vi "Run.vi"(8 "error in (no error)":errorcluster, 11 "SecMirror in":refnum<class "SecMirror.lvclass">) -> (0 "error out":errorcluster, 3 "SecMirror out":refnum<class "SecMirror.lvclass">)   [LabVIEW 2018, in "SecMirror.lvclass"]
uses:
  SecMirror.lvclass
  SecMirror.lvclass/SecMirror.ctl
  Device/Device.lvclass
  StateMachine/State Machine.lvclass
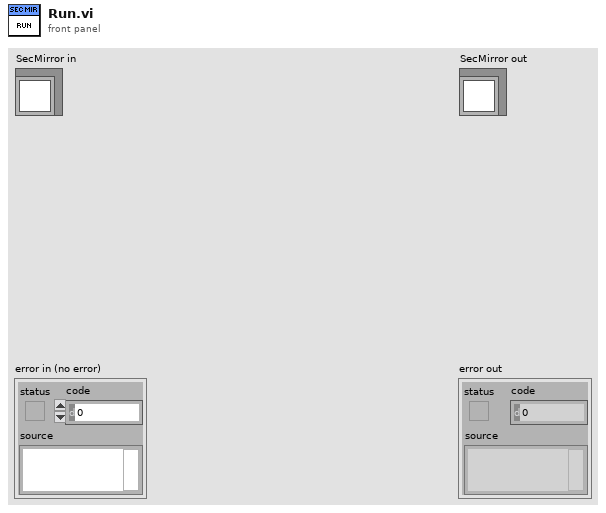
[diagram p1: front panel]
types:
  T1 = cluster{"clientId":string, "clientTransactionId":string, "clientName":string, "action":string}
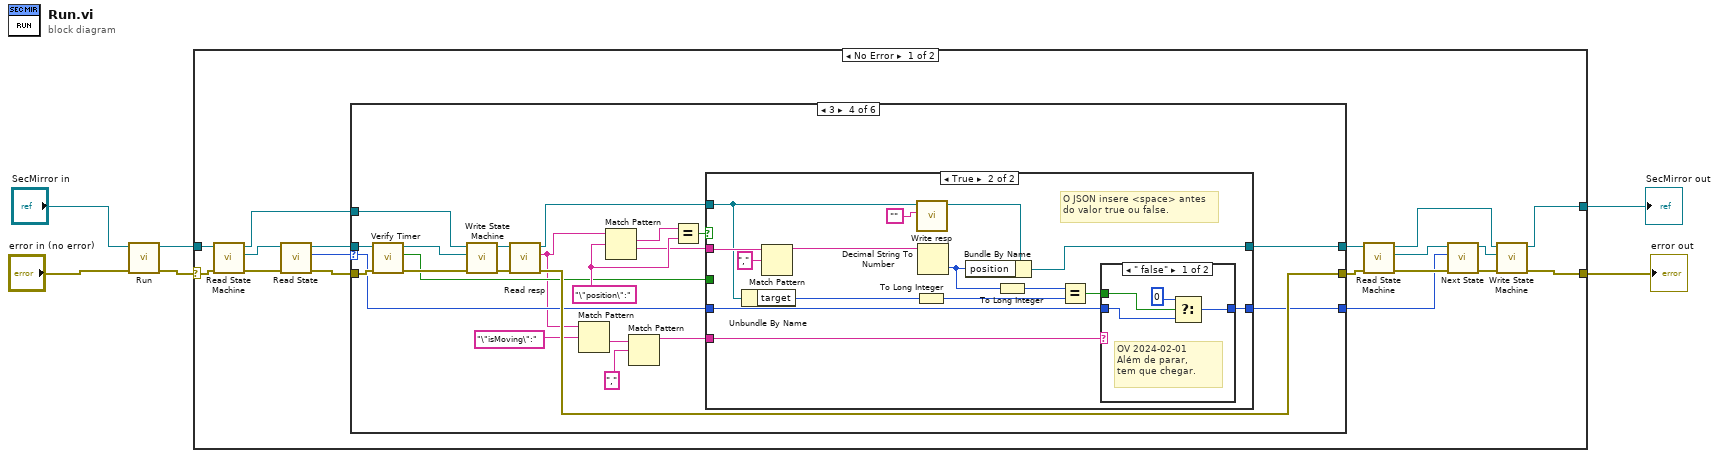
[diagram p0: block diagram]
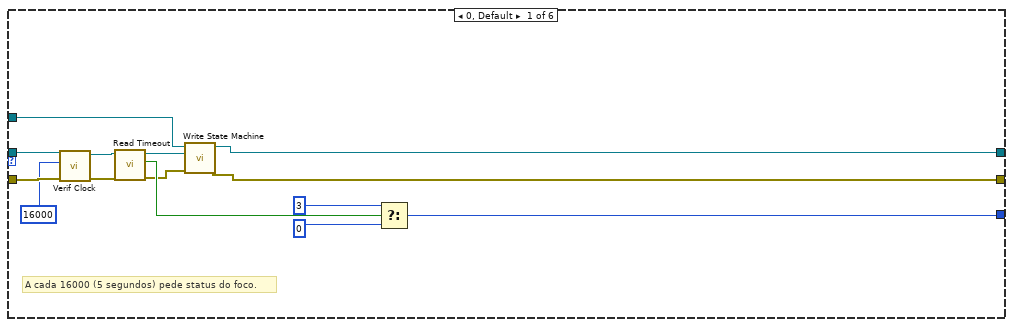
[diagram p2: hidden frame]
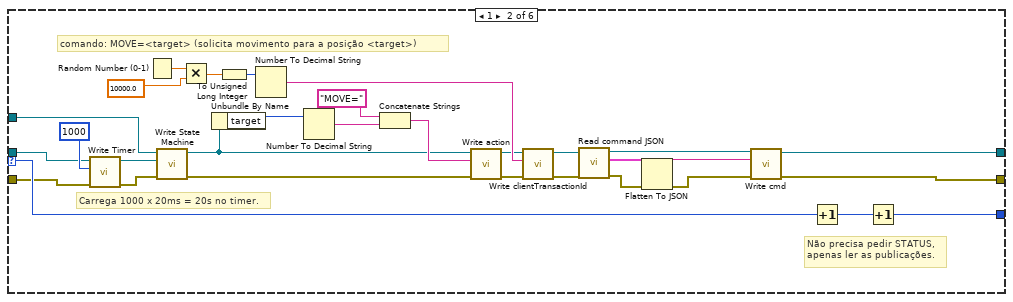
[diagram p3: hidden frame]
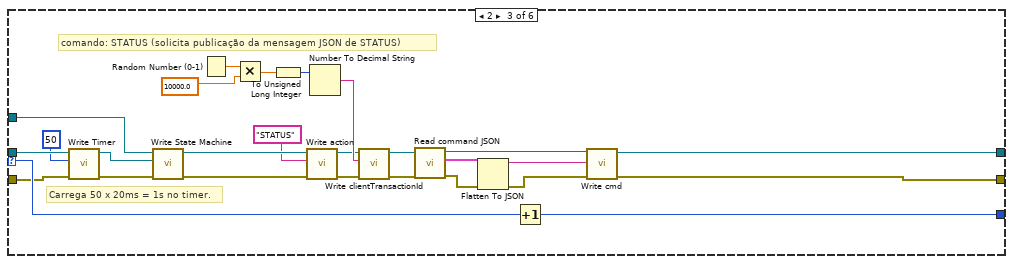
[diagram p4: hidden frame]
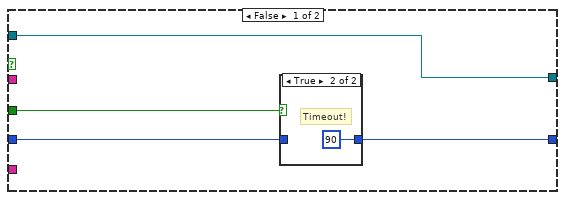
[diagram p5: hidden frame]
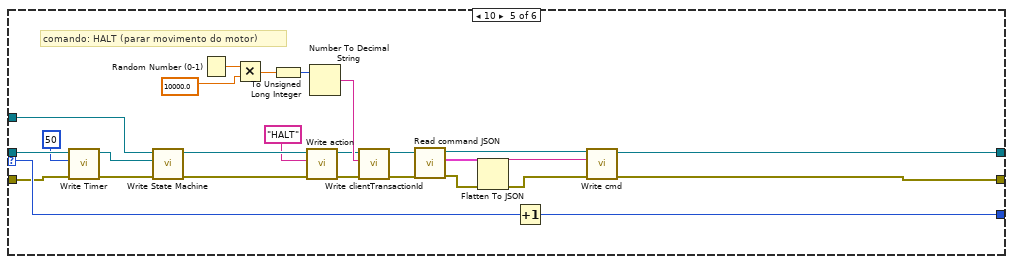
[diagram p8: hidden frame]
diagram:
  n1 = call-parent "Run.vi"("error in (no error)"="error in (no error)", "Device in"="SecMirror in") -> ("error out"=w3:errorcluster, "Device out"=w4:refnum<class "SecMirror.lvclass">)  [unwired: 8 in]
  n2 = case shown="No Error" w3 {
    selector: w3 -> [w23 w176]
    tunnel: [w15 w176] -> w1
    tunnel: w4 -> [w24 w175]
    tunnel: [w14 w175] -> w2
    frame No Error {
      n3 = call-dynamic "Read State Machine.vi"("error in (no error)"=w23, "Device in"=w24) -> ("error out"=w21:errorcluster, "State Machine.lvclass"=w22:refnum<class "State Machine.lvclass">, "Device out"=w12:refnum<class "SecMirror.lvclass">)  [unwired: 7 in]
      n4 = call-dynamic "Read State.vi"("error in (no error)"=w21, "State Machine in"=w22) -> ("error out"=w11:errorcluster, "State"=w13:i32, "State Machine out"=w7:refnum<class "State Machine.lvclass">)  [unwired: 7 in]
      n5 = case shown="3" w13 {
        selector: w13 -> [_ w69 w96 w107 w171 w172]
        tunnel: w12 -> [w30 w46 w92 w112 w167 w174]
        tunnel: w11 -> [w33 w44 w91 w110 w166 w173]
        tunnel: [w26 w39 w70 w116 w145 w173] -> w10
        tunnel: [w27 w40 w71 w117 w146 w174] -> w9
        tunnel: [w38 w49 w95 w115 w170 w172] -> w8
        tunnel: w7 -> [w32 w47 w94 w114 w169 _]
        frame 0, Default {
          # "A cada 16000 (5 segundos) pede status do foco."
          n6 = call-dynamic "Verif Clock.vi"("error in (no error)"=w33, "period (ms)"=u32 16000 ("period"), "State Machine in"=w32) -> ("error out"=w34:errorcluster, "State Machine out"=w31:refnum<class "State Machine.lvclass">)  [unwired: 6 in, 1 out]
          n7 = call-dynamic "Read Timeout.vi"("error in (no error)"=w34, "State Machine in"=w31) -> ("error out"=w28:errorcluster, "Timeout"=w35:bool, "State Machine out"=w29:refnum<class "State Machine.lvclass">)  [unwired: 7 in]
          n8 = call-dynamic "Write State Machine.vi"("error in (no error)"=w28, "State Machine.lvclass"=w29, "Device in"=w30) -> ("error out"=w26:errorcluster, "Device out"=w27:refnum<class "SecMirror.lvclass">)  [unwired: 7 in]
          n9 = Select(t=3 ("State"), s=w35, f=0 ("State")) -> (s? t:f=w38:i32)
        }
        frame 1 {
          # "Carrega 1000 x 20ms = 20s no timer."
          # "Não precisa pedir STATUS,\napenas ler as publicações."
          # "comando: MOVE=<target> (solicita movimento para a posição <target>)"
          n10 = call-dynamic "Write Timer.vi"("error in (no error)"=w44, "Timer"=u32 1000, "State Machine in"=w47) -> ("error out"=w43:errorcluster, "State Machine out"=w42:refnum<class "State Machine.lvclass">)  [unwired: 7 in]
          n11 = Random Number (0-1)() -> (number: 0 to 1=w64:dbl)
          n12 = call-dynamic "Write State Machine.vi"("error in (no error)"=w43, "State Machine.lvclass"=w42, "Device in"=w46) -> ("error out"=w41:errorcluster, "Device out"=w45:refnum<class "SecMirror.lvclass">)  [unwired: 7 in]
          n13 = Multiply(x=w64, y=10000.0) -> (x*y=w61:dbl)
          n14 = Unbundle By Name(w45) -> ("target"=w66:i32)
          n15 = To Unsigned Long Integer(number=w61) -> (unsigned 32bit integer=w60:u32)
          n16 = Number To Decimal String(number=w60) -> (decimal integer string=w59:string)  [unwired: 1 in]
          n17 = Number To Decimal String(number=w66) -> (decimal integer string=w65:string)  [unwired: 1 in]
          n18 = Concatenate Strings("MOVE=" ("cmd"), w65) -> (w63:string)
          n19 = call-dynamic "Write action.vi"("error in (no error)"=w41, "action"=w63, "Device in"=w45) -> ("error out"=w57:errorcluster, "Device out"=w58:refnum<class "SecMirror.lvclass">)  [unwired: 7 in]
          n20 = call-dynamic "Write clientTransactionId.vi"("error in (no error)"=w57, "clientTransactionId"=w59, "Device in"=w58) -> ("error out"=w55:errorcluster, "Device out"=w56:refnum<class "SecMirror.lvclass">)  [unwired: 7 in]
          n21 = call-dynamic "Read command JSON.vi"("error in (no error)"=w55, "Device in"=w56) -> ("error out"=w53:errorcluster, "command JSON"=w54:T1, "Device out"=w52:refnum<class "SecMirror.lvclass">)  [unwired: 7 in]
          n22 = Flatten To JSON(anything=w54, error in (no error)=w53) -> (JSON string=w50:string, 11:w51:errorcluster)  [unwired: 1 in]
          n23 = call-dynamic "Write cmd.vi"("error in (no error)"=w51, "cmd"=w50, "Device in"=w52) -> ("error out"=w39:errorcluster, "Device out"=w40:refnum<class "SecMirror.lvclass">)  [unwired: 7 in]
          n24 = Increment(x=w69) -> (x+1=w68:i32)
          n25 = Increment(x=w68) -> (x+1=w49:i32)
        }
        frame 2 {
          # "Carrega 50 x 20ms = 1s no timer."
          # "comando: STATUS (solicita publicação da mensagem JSON de STATUS)"
          n26 = call-dynamic "Write Timer.vi"("error in (no error)"=w91, "Timer"=u32 50, "State Machine in"=w94) -> ("error out"=w90:errorcluster, "State Machine out"=w89:refnum<class "State Machine.lvclass">)  [unwired: 7 in]
          n27 = call-dynamic "Write State Machine.vi"("error in (no error)"=w90, "State Machine.lvclass"=w89, "Device in"=w92) -> ("error out"=w74:errorcluster, "Device out"=w73:refnum<class "SecMirror.lvclass">)  [unwired: 7 in]
          n28 = Random Number (0-1)() -> (number: 0 to 1=w88:dbl)
          n29 = Multiply(x=w88, y=10000.0) -> (x*y=w86:dbl)
          n30 = To Unsigned Long Integer(number=w86) -> (unsigned 32bit integer=w85:u32)
          n31 = call-dynamic "Write action.vi"("error in (no error)"=w74, "action"="STATUS" ("cmd"), "Device in"=w73) -> ("error out"=w82:errorcluster, "Device out"=w83:refnum<class "SecMirror.lvclass">)  [unwired: 7 in]
          n32 = Number To Decimal String(number=w85) -> (decimal integer string=w84:string)  [unwired: 1 in]
          n33 = call-dynamic "Write clientTransactionId.vi"("error in (no error)"=w82, "clientTransactionId"=w84, "Device in"=w83) -> ("error out"=w80:errorcluster, "Device out"=w81:refnum<class "SecMirror.lvclass">)  [unwired: 7 in]
          n34 = call-dynamic "Read command JSON.vi"("error in (no error)"=w80, "Device in"=w81) -> ("error out"=w78:errorcluster, "command JSON"=w79:T1, "Device out"=w77:refnum<class "SecMirror.lvclass">)  [unwired: 7 in]
          n35 = Flatten To JSON(anything=w79, error in (no error)=w78) -> (JSON string=w75:string, 11:w76:errorcluster)  [unwired: 1 in]
          n36 = Increment(x=w96) -> (x+1=w95:i32)
          n37 = call-dynamic "Write cmd.vi"("error in (no error)"=w76, "cmd"=w75, "Device in"=w77) -> ("error out"=w70:errorcluster, "Device out"=w71:refnum<class "SecMirror.lvclass">)  [unwired: 7 in]
        }
        frame 3 {
          w104 = "\"position\":" ("regular expression")
          n38 = call "Verify Timer.vi"("error in (no error)"=w110, "State Machine in"=w114) -> ("error out"=w111:errorcluster, "timeout"=w103:bool, "State Machine out"=w113:refnum<class "State Machine.lvclass">)  [unwired: 7 in]
          n39 = call-dynamic "Write State Machine.vi"("error in (no error)"=w111, "State Machine.lvclass"=w113, "Device in"=w112) -> ("error out"=w108:errorcluster, "Device out"=w109:refnum<class "SecMirror.lvclass">)  [unwired: 7 in]
          n40 = call-dynamic "Read resp.vi"("error in (no error)"=w108, "Device in"=w109) -> ("error out"=w116:errorcluster, "resp"=w101:string, "Device out"=w118:refnum<class "SecMirror.lvclass">)  [unwired: 7 in]
          n41 = Match Pattern(string=w101, regular expression="\"isMoving\":") -> (after substring=w98:string)  [unwired: 1 in, 3 out]
          n42 = Match Pattern(string=w101, regular expression=w104) -> (match substring=w105:string, after substring=w102:string)  [unwired: 1 in, 2 out]
          n43 = Match Pattern(string=w98, regular expression=",") -> (before substring=w97:string)  [unwired: 1 in, 3 out]
          n44 = Equal?(x=w105, y=w104) -> (x = y?=w106:bool)
          n45 = case shown="True" w106 {
            tunnel: w118 -> [w122 w130]
            tunnel: [w122 w138] -> w117
            tunnel: [w120 w139] -> w115
            tunnel: w107 -> [w121 w131]
            tunnel: w103 -> [w119 _]
            tunnel: w102 -> [_ w134]
            tunnel: w97 -> [_ w132]
            frame False {
              n46 = case shown="True" w119 {
                tunnel: w121 -> [w123 _]
                tunnel: [w123 90 ("State")] -> w120
                frame False {
                }
                frame True {
                  # "Timeout!"
                }
              }
            }
            frame True {
              # "O JSON insere <space> antes\ndo valor true ou false."
              n47 = Unbundle By Name(w130) -> ("target"=w128:i32)
              n48 = Match Pattern(string=w134, regular expression=",") -> (before substring=w133:string)  [unwired: 1 in, 3 out]
              n49 = To Long Integer(number=w128) -> (32bit integer=w125:i32)
              n50 = call-dynamic "Write resp.vi"("resp"="", "Device in"=w130) -> ("Device out"=w137:refnum<class "SecMirror.lvclass">)  [unwired: 8 in, 1 out]
              n51 = Decimal String To Number(string=w133) -> (number=w129:i32)  [unwired: 2 in, 1 out]
              n52 = Bundle By Name(cluster=w137, "position"=w129) -> (w138:refnum<class "SecMirror.lvclass">)
              n53 = To Long Integer(number=w129) -> (32bit integer=w126:i32)
              n54 = Equal?(x=w126, y=w125) -> (x = y?=w127:bool)
              n55 = case shown="\" false\"" w132 {
                tunnel: [w140 w144] -> w139
                tunnel: w131 -> [w141 w144]
                tunnel: w127 -> [w142 _]
                frame " false" {
                  # "OV 2024-02-01\nAlém de parar,\ntem que chegar."
                  n56 = Select(t=0, s=w142, f=w141) -> (s? t:f=w140:i32)
                }
                frame " true", Default {
                }
              }
            }
          }
        }
        frame 10 {
          # "comando: HALT (parar movimento do motor)"
          n57 = call-dynamic "Write Timer.vi"("error in (no error)"=w166, "Timer"=u32 50, "State Machine in"=w169) -> ("error out"=w165:errorcluster, "State Machine out"=w164:refnum<class "State Machine.lvclass">)  [unwired: 7 in]
          n58 = call-dynamic "Write State Machine.vi"("error in (no error)"=w165, "State Machine.lvclass"=w164, "Device in"=w167) -> ("error out"=w149:errorcluster, "Device out"=w148:refnum<class "SecMirror.lvclass">)  [unwired: 7 in]
          n59 = Random Number (0-1)() -> (number: 0 to 1=w163:dbl)
          n60 = Multiply(x=w163, y=10000.0) -> (x*y=w161:dbl)
          n61 = To Unsigned Long Integer(number=w161) -> (unsigned 32bit integer=w160:u32)
          n62 = call-dynamic "Write action.vi"("error in (no error)"=w149, "action"="HALT" ("cmd"), "Device in"=w148) -> ("error out"=w157:errorcluster, "Device out"=w158:refnum<class "SecMirror.lvclass">)  [unwired: 7 in]
          n63 = Number To Decimal String(number=w160) -> (decimal integer string=w159:string)  [unwired: 1 in]
          n64 = call-dynamic "Write clientTransactionId.vi"("error in (no error)"=w157, "clientTransactionId"=w159, "Device in"=w158) -> ("error out"=w155:errorcluster, "Device out"=w156:refnum<class "SecMirror.lvclass">)  [unwired: 7 in]
          n65 = call-dynamic "Read command JSON.vi"("error in (no error)"=w155, "Device in"=w156) -> ("error out"=w153:errorcluster, "command JSON"=w154:T1, "Device out"=w152:refnum<class "SecMirror.lvclass">)  [unwired: 7 in]
          n66 = Flatten To JSON(anything=w154, error in (no error)=w153) -> (JSON string=w150:string, 11:w151:errorcluster)  [unwired: 1 in]
          n67 = Increment(x=w171) -> (x+1=w170:i32)
          n68 = call-dynamic "Write cmd.vi"("error in (no error)"=w151, "cmd"=w150, "Device in"=w152) -> ("error out"=w145:errorcluster, "Device out"=w146:refnum<class "SecMirror.lvclass">)  [unwired: 7 in]
        }
        frame 90 {
          # "Situacao de erro: O focalizador do 1.60 nao publicou o STATUS por 100 x 20m = 2s (estado 1)"
        }
      }
      n69 = call-dynamic "Read State Machine.vi"("error in (no error)"=w10, "Device in"=w9) -> ("error out"=w17:errorcluster, "State Machine.lvclass"=w19:refnum<class "State Machine.lvclass">, "Device out"=w18:refnum<class "SecMirror.lvclass">)  [unwired: 7 in]
      n70 = call "Next State.vi"("error in (no error)"=w17, "New_State"=w8, "State Machine in"=w19) -> ("error out"=w16:errorcluster, "State Machine out"=w20:refnum<class "State Machine.lvclass">)  [unwired: 7 in]
      n71 = call-dynamic "Write State Machine.vi"("error in (no error)"=w16, "State Machine.lvclass"=w20, "Device in"=w18) -> ("error out"=w15:errorcluster, "Device out"=w14:refnum<class "SecMirror.lvclass">)  [unwired: 7 in]
    }
    frame Error {
    }
  }
  "error out" <- w1
  "SecMirror out" <- w2
